vi "TCP Multiple Connections - Client 1.vi"() -> ()   [LabVIEW 2013]
doc: "建立TCP Multiple Connections - Server.vi的连接。单击“停止”按钮后，VI发送单个字符通知服务器VI断开连接。"
panel:
  in  "服务器关闭":string="服务器VI关闭了连接。"
  out "服务器数据":dbl(graph)
  in  "停止":bool
  # "概述：演示使用TCP函数连接至正在向多个客户端VI发送数据的TCP服务器VI。\n操作步骤：\n1. 确保已运行TCP Multiple Connections - Server.vi。\n2. 运行VI。\n3. 注意服务器数据图表开始更新，服务器VI上客户端连接数量的值以1递增。\n4. 单击停止可停止VI。注意，服务器VI上“客户端连接数量”的值以1递减。"
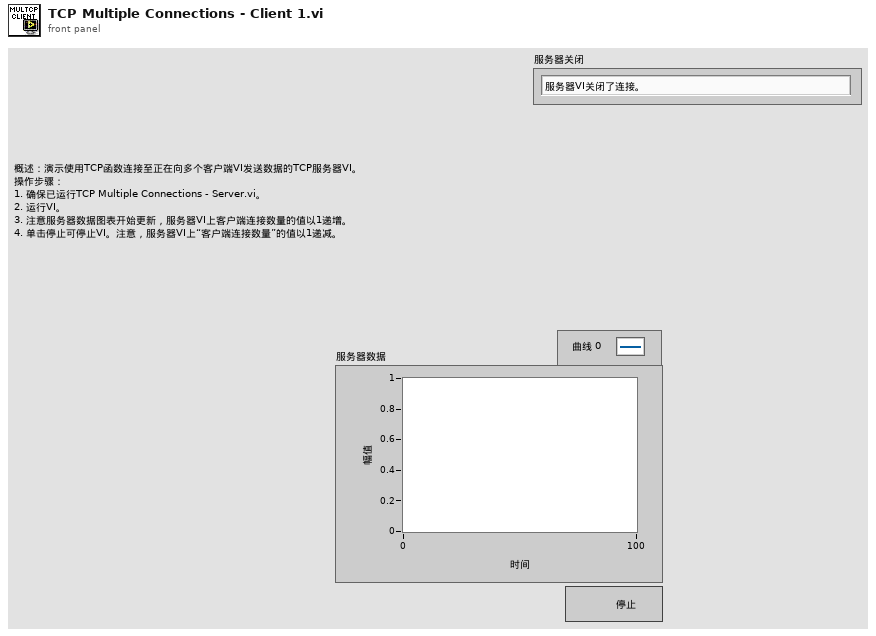
[diagram p1: front panel]
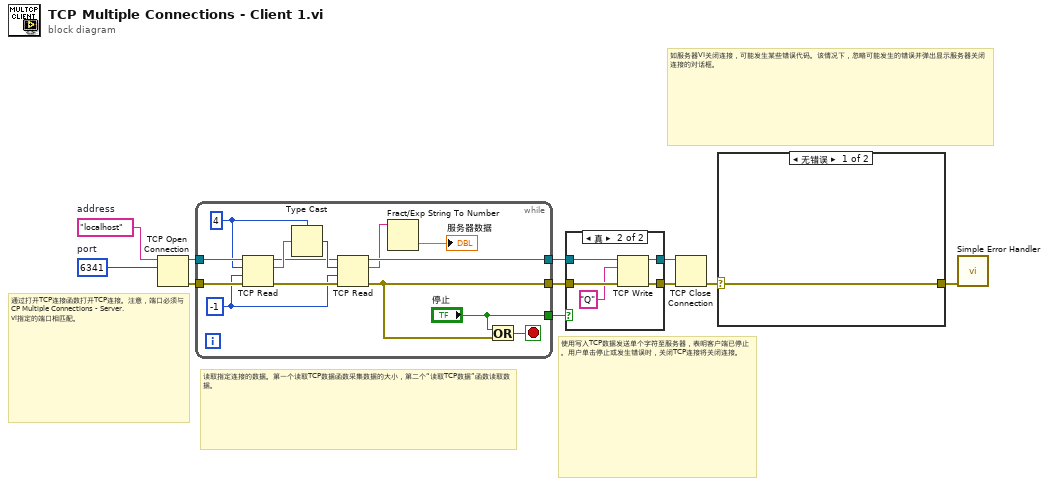
[diagram p0: block diagram]
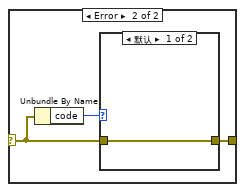
[diagram p2: hidden frame]
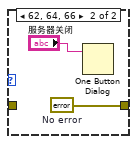
[diagram p3: hidden frame]
diagram:
  w10 = u16 6341  # port
  w11 = "localhost"  # address
  # "如服务器VI关闭连接，可能发生某些错误代码。该情况下，忽略可能发生的错误并弹出显示服务器关闭连接的对话框。"
  # "使用写入TCP数据发送单个字符至服务器，表明客户端已停止。用户单击停止或发生错误时，关闭TCP连接将关闭连接。"
  # "读取指定连接的数据。第一个读取TCP数据函数采集数据的大小，第二个“读取TCP数据”函数读取数据。"
  # "通过打开TCP连接函数打开TCP连接。注意，端口必须与CP Multiple Connections - Server.vi指定的端口相匹配。"
  n1 = TCP Open Connection(address=w11, remote port or service name=w10) -> (connection ID=w9:refnum<k5>, error out=w8:errorcluster)  [unwired: 1 in, 2 out]
  n2 = while {
    tunnel: ["停止"] -> w3
    tunnel: [w19] -> w7
    tunnel: [w16] -> w5
    tunnel: w8 -> [w24]
    tunnel: w9 -> [w25]
    stop <- w18 stop-if-true
    w12 = -1
    w13 = 4
    n3 = TCP Read(connection ID=w25, bytes to read=w13, error in (no error)=w24, 9:w12) -> (connection ID out=w20:refnum<k5>, data out=w23:string, error out=w22:errorcluster)  [unwired: 1 out]
    n4 = Type Cast(type=w13, x=w23) -> (*(type *) &x=w21:i32)
    n5 = TCP Read(connection ID=w20, bytes to read=w21, error in (no error)=w22, 9:w12) -> (connection ID out=w19:refnum<k5>, data out=w15:string, error out=w16:errorcluster)  [unwired: 1 out]
    n6 = Fract/Exp String To Number(string=w15) -> (number=→"服务器数据":dbl)  [unwired: 3 in, 1 out]
    n7 = Or(x="停止", y=w16) -> (x .or. y?=w18:bool)
  }
  n8 = case shown="真" w3 {
    tunnel: w7 -> [w27 w32]
    tunnel: [w27 w30] -> w6
    tunnel: w5 -> [w26 w31]
    tunnel: [w26 w29] -> w4
    frame False {
    }
    frame True {
      n9 = TCP Write(connection ID=w32, data in="Q", error in (no error)=w31) -> (connection ID out=w30:refnum<k5>, error out=w29:errorcluster)  [unwired: 2 out]
    }
  }
  n10 = TCP Close Connection(connection ID=w6, error in (no error)=w4) -> (error out=w2:errorcluster)  [unwired: 2 out]
  n11 = case shown="无错误" w2 {
    selector: w2 -> [w33 w35]
    tunnel: [w33 w34] -> w1
    frame No Error {
    }
    frame Error {
      n12 = Unbundle By Name(w35) -> ("code"=w36:i32)
      n13 = case shown="默认" w36 {
        tunnel: w35 -> [w37 _]
        tunnel: [w37 w39] -> w34
        frame Default {
        }
        frame 62, 64, 66 {
          w39 = errorcluster {"status"=FALSE, "code"=0, "source"=""}  # No error
          n14 = One Button Dialog(message="服务器关闭") -> ()  [unwired: 1 in, 1 out]
        }
      }
    }
  }
  n15 = call <vilib>:"Simple Error Handler.vi"("error in (no error)"=w1) -> ()  [unwired: 1 in, 8 out]
